vi "logic-train-sample-7-1-drum-seq.vi"(9 "Cancel":bool, 11 "Request\nCapture":bool) -> (0 "Seq  Active":bool, 1 "Ready":bool, 2 "Hand_Close":bool, 3 "Arm_Extend":bool, 4 "Error":bool, 5 "Step Number":T1=enum."Initialize")   [LabVIEW 2020]
uses:
  <vilib>/Rock Robotics/WPI/ThirdParty/JAS_Junk/TrajLib/Enum/DrumSequence_Step_Enum.ctl
  <vilib>/Rock Robotics/WPI/ThirdParty/JAS_Junk/TrajLib/Timer_New.vi
  <vilib>/Rock Robotics/WPI/ThirdParty/JAS_Junk/TrajLib/VI/DigSeqLogic_Edge_On.vi
  <vilib>/Rock Robotics/WPI/ThirdParty/JAS_Junk/TrajLib/Util_GetTime.vi
  <vilib>/Rock Robotics/WPI/ThirdParty/JAS_Junk/TrajLib/VI/Util_GetTime_U32.vi
  <vilib>/Utility/semaphor.llb/Obtain Semaphore Reference.vi
  <vilib>/Rock Robotics/WPI/ThirdParty/JAS_Junk/TrajLib/Timer_Reset.vi
  <vilib>/Rock Robotics/WPI/ThirdParty/JAS_Junk/TrajLib/Timer_Start.vi
  <vilib>/Rock Robotics/WPI/ThirdParty/JAS_Junk/TrajLib/Timer_Stop.vi
  <vilib>/Rock Robotics/WPI/ThirdParty/JAS_Junk/TrajLib/Timer_HasPeriodPassedOnce.vi
  <vilib>/Rock Robotics/WPI/ThirdParty/JAS_Junk/TrajLib/VI/Util_GetTime_U64.vi
  <vilib>/Rock Robotics/WPI/ThirdParty/JAS_Junk/TrajLib/VI/Timer_Restart.vi
  <vilib>/Rock Robotics/WPI/ThirdParty/JAS_Junk/TrajLib/Trajectory_Library.lvlib
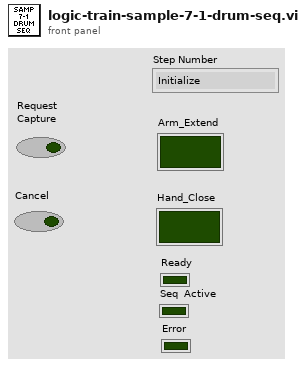
[diagram p1: front panel]
types:
  T1 = typedef "Trajectory_Library.lvlib/DrumSequence_Step_Enum.ctl" = enum16{"Do Nothing", "Step 1", "Step 2", "Step 3", "Step 4", "Step 5", "Step 6", "Step 7", "Step 8", "Step 9", "Step 10", "Step 11", "Step 12", "Step 13", "Step 14", "Step 15", "Step 16", "Step 17", "Step 18", "Step 19", "Step 20", "Step 21", "Step 22", "Step 23", "Step 24", "Step 25", "Step 26", "Step 27", "Step 28", "Step 29", "Step 30", "Step 31", "Step 32", "Cancel", "Initialize", "Error"}
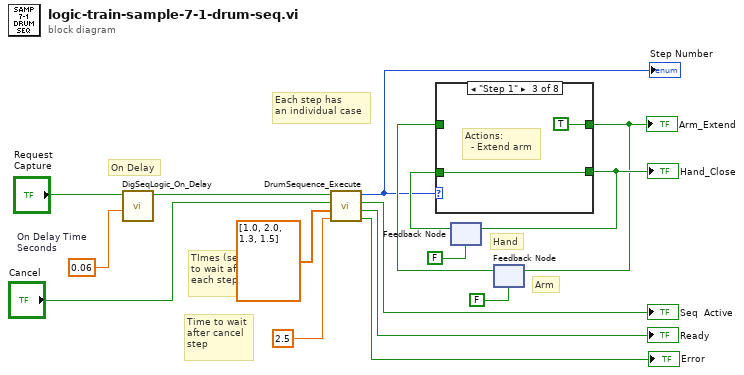
[diagram p0: block diagram]
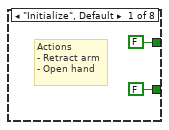
[diagram p2: hidden frame]
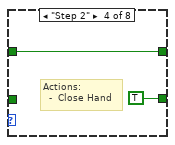
[diagram p4: hidden frame]
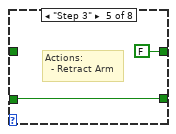
[diagram p5: hidden frame]
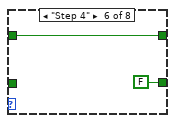
[diagram p6: hidden frame]
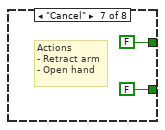
[diagram p7: hidden frame]
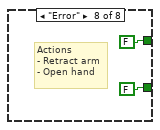
[diagram p8: hidden frame]
diagram:
  w10 = 0.06  # On Delay Time Seconds
  # "Time to wait\nafter cancel\nstep"
  # "TImes (sec)\nto wait after\neach step"
  # "Each step has\nan individual case"
  # "On Delay"
  # "Arm"
  # "Hand"
  n1 = call <vilib>:"DigSeqLogic_On_Delay.vi"("Delay"=w10, "Input"="Request\nCapture") -> ("Output"=w8:bool)  [unwired: 8 in, 1 out]
  n2 = call <vilib>:"DrumSequence_Execute.vi"("Cancel Time Sec"=2.5, "Step Times Sec"=dbl[] [1.0, 2.0, 1.3, 1.5], "Cancel"="Cancel", "Initiate"=w8) -> ("Error"=→"Error":bool, "Ready"=→"Ready":bool, "Seq  Active"=→"Seq  Active":bool, "Step Number"=w6:T1)  [unwired: 4 in]
  "Step Number" <- w6
  n3 = feedback #1(FALSE) -> (w12:bool)
  n4 = feedback #2(FALSE) -> (w11:bool)
  n5 = case shown="\"Step 1\"" w6 {
    tunnel: [FALSE w20 TRUE w24 FALSE w28 FALSE FALSE] -> w15
    tunnel: [FALSE w19 w21 TRUE w25 FALSE FALSE FALSE] -> w16
    tunnel: w12 -> [_ w19 w21 _ w25 _ _ _]
    tunnel: w11 -> [_ w20 _ w24 _ w28 _ _]
    frame "Initialize", Default {
      # "Actions\n- Retract arm\n- Open hand"
    }
    frame "Do Nothing" {
    }
    frame "Step 1" {
      # "Actions:\n  - Extend arm"
    }
    frame "Step 2" {
      # "Actions:\n  -  Close Hand"
    }
    frame "Step 3" {
      # "Actions:\n  - Retract Arm"
    }
    frame "Step 4" {
    }
    frame "Cancel" {
      # "Actions\n- Retract arm\n- Open hand"
    }
    frame "Error" {
      # "Actions\n- Retract arm\n- Open hand"
    }
  }
  "Arm_Extend" <- w15
  "Hand_Close" <- w16
  n6 = feedback-in #1(w16) -> ()
  n7 = feedback-in #2(w15) -> ()
